vi "BRig_Host_dataRunState_dataPlot_wrong3.vi"() -> (2 "output_idx_dataPlot_wrong3":i32)   [LabVIEW 2014]
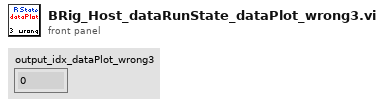
[diagram p1: front panel]
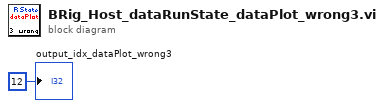
[diagram p0: block diagram]
diagram:
  "output_idx_dataPlot_wrong3" <- 12 ("output_idx_dataTS")
